vi "FR GUI Recalculate.vi"(11 "FFmeter settings":T1={"AC Source"={"AC Source type"=enum."Fluke 5XXX calibrator", "VISA"="", "Ref. clock (Hz)"=0.0, "status ref"=refnum}, "TWM pipe"="\\\\.\\pipe\\TWM:server", "Measurement status ref"=refnum, "TWM Status ref"=refnum, "Abort ref"=refnum, "DC meter"={"DC meter type"=enum."H/A/K 3458", "DC meter VISA"="", "NPLC"=10, "status ref"=refnum}, "Measurement properties"={"Measurement frequencies (Hz)"=[1000.0], "Sampling frequency (Hz)"=500000.0, "Signal amplitude (V)"=4.5, "AC-DC settle time (s)"=20.0, "Record length (multiples of period)"=[1000.0, 10000.0, 1000.0], "Measurement template file"=path "", "Row of START keyword"=0, "Row of STOP keyword"=0, "Calculate RMS from samples"=FALSE, "AC-DC warm up time (s)"=300.0, "Measurement template line"=[], "DC meter readings No."=10, "Algorithm"="TWM-WFFT", "Simultaneous measurement"=FALSE}, "Skip waiting ref"=refnum, "Octave paths"={"GNU Octave path"=path "C:/Program Files/GNU Octave/Octave-6.2.0/mingw64/bin", "TWM+QWTB path"=path "C:/Users/labina/Desktop/TWM-1.8.7.0-full/octprog", "lvlib path"=path "D:/martin/WAC/WACsw - github/control_software/Filter function meter/external libraries/GOLPI 0.7.3.1 source distribution LV 20.0 32 bit/lv_proc.dll"}, "Template definition"={"Keywords column"=0, "Sig. freq. column"=1, "Rec. len. column"=2, "Meas. points. row min to read"=9, "Meas. points. row max to read"=1509, "Properties column"=4, "Properties row start"=1, "Properties row end"=5, "Keyword START regexp"="", "Keyword STOP regexp"="", "HW data column"=7, "HW data row start"=1, "HW data row end"=3, "TIme and date column start"=3, "Digitizer value column start "=4, "DC mean column start "=6, "DC readings column start"=10}} {"Measurement properties"."Record length (multiples of period)" format="%#_3p"; "Measurement properties"."Sampling frequency (Hz)" format="%#_3p"; "Measurement properties"."Measurement frequencies (Hz)" format="%#_3p"}) -> (3 "FFmeter settings out":T1={"AC Source"={"AC Source type"=enum."Fluke 5XXX calibrator", "VISA"="", "Ref. clock (Hz)"=0.0, "status ref"=refnum}, "TWM pipe"="\\\\.\\pipe\\TWM:server", "Measurement status ref"=refnum, "TWM Status ref"=refnum, "Abort ref"=refnum, "DC meter"={"DC meter type"=enum."H/A/K 3458", "DC meter VISA"="", "NPLC"=10, "status ref"=refnum}, "Measurement properties"={"Measurement frequencies (Hz)"=[1000.0], "Sampling frequency (Hz)"=500000.0, "Signal amplitude (V)"=4.5, "AC-DC settle time (s)"=20.0, "Record length (multiples of period)"=[1000.0, 10000.0, 1000.0], "Measurement template file"=path "", "Row of START keyword"=0, "Row of STOP keyword"=0, "Calculate RMS from samples"=FALSE, "AC-DC warm up time (s)"=300.0, "Measurement template line"=[], "DC meter readings No."=10, "Algorithm"="TWM-WFFT", "Simultaneous measurement"=FALSE}, "Skip waiting ref"=refnum, "Octave paths"={"GNU Octave path"=path "C:/Program Files/GNU Octave/Octave-6.2.0/mingw64/bin", "TWM+QWTB path"=path "C:/Users/labina/Desktop/TWM-1.8.7.0-full/octprog", "lvlib path"=path "D:/martin/WAC/WACsw - github/control_software/Filter function meter/external libraries/GOLPI 0.7.3.1 source distribution LV 20.0 32 bit/lv_proc.dll"}, "Template definition"={"Keywords column"=0, "Sig. freq. column"=1, "Rec. len. column"=2, "Meas. points. row min to read"=9, "Meas. points. row max to read"=1509, "Properties column"=4, "Properties row start"=1, "Properties row end"=5, "Keyword START regexp"="", "Keyword STOP regexp"="", "HW data column"=7, "HW data row start"=1, "HW data row end"=3, "TIme and date column start"=3, "Digitizer value column start "=4, "DC mean column start "=6, "DC readings column start"=10}} {"Measurement properties"."Record length (multiples of period)" format="%#_3p"; "Measurement properties"."Sampling frequency (Hz)" format="%#_3p"; "Measurement properties"."Measurement frequencies (Hz)" format="%#_3p"})   [LabVIEW 2020]
doc: "Use this template to build a producer/consumer design pattern with events to produce queue items. Use this design pattern instead of the User Interface Event Handler pattern for user interfaces when you want to execute code asynchronously in response to an event without slowing the user interface responsiveness."
uses:
  Type definitions/FFmeter settings.ctl
  General AC source/Type definitions/AC Source.ctl
  General AC source/Type definitions/AC Source type.ctl
  General DC meter/Type definitions/DC meter.ctl
  General DC meter/Type definitions/DC meter type.ctl
  FR Measurement/Type definitions/FR Measuement properties.ctl
  FR Utilities/Type definitions/FR Template definition.ctl
  <vilib>/Utility/NIReport.llb/Report Type.ctl
  external libraries/GOLPI 0.7.3.1 source distribution LV 20.0 32 bit/GOLPI reference Type Def.ctl
  external libraries/GOLPI 0.7.3.1 source distribution LV 20.0 32 bit/Pipe Handle.ctl
  <vilib>/Utility/error.llb/Error Cluster From Error Code.vi
  <vilib>/addons/_office/excel.llb/Excel Get Data ([str]).vi
  <vilib>/ErrorRing/Error Ring.xnode
  <vilib>/Utility/NIReport.llb/NI_report.lvclass
  external libraries/varilib/varilib.lvlib
  <vilib>/addons/_office/NI_ReportGenerationToolkit.lvlib
  <vilib>/Utility/NIReport.llb/NI_ReportGenerationCore.lvlib
  external libraries/GOLPI 0.7.3.1 source distribution LV 20.0 32 bit/LV Process library.lvlib
  external libraries/GOLPI 0.7.3.1 source distribution LV 20.0 32 bit/GOLPI library.lvlib
  <vilib>/Utility/NIReport.llb/Excel/NI_Excel.lvclass
panel:
  out "template file":string
  in  "Abort":bool
  in  "skip calculated":bool caption="Skip already calculated (only rereads results)"
  out "Progress":i32(slide) min=0 max=266 scale=0.0..10.0
  in  "TWM+QWTB path":path=path "C:/Users/labina/Desktop/TWM-1.8.7.0-full/octprog"
  in  "GNU Octave path":path=path "C:/Program Files/GNU Octave/Octave-6.2.0/mingw64/bin"
  out "gui_elements":refnum<vi>[](array[refnum])
  in  "OK":bool
  in  "cancel":bool
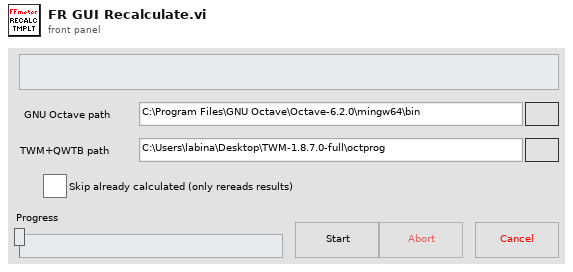
[diagram p1: front panel]
types:
  T1 = typedef "FFmeter settings.ctl" = cluster{"AC Source":T2, "TWM pipe":string, "Measurement status ref":refnum<vi>, "TWM Status ref":refnum<vi>, "Abort ref":refnum<vi>, "DC meter":T4, "Measurement properties":T6, "Skip waiting ref":refnum<vi>, "Octave paths":cluster{"GNU Octave path":path, "TWM+QWTB path":path, "lvlib path":path}, "Template definition":T7}
  T2 = typedef "AC Source.ctl" = cluster{"AC Source type":T3, "VISA":refnum<visa-resource-name>, "Ref. clock (Hz)":dbl, "status ref":refnum<vi>}
  T3 = typedef "AC Source type.ctl" = enum16{"Fluke 5XXX calibrator", "Tektronix AFG3000 series", "dummy"}
  T4 = typedef "DC meter.ctl" = cluster{"DC meter type":T5, "DC meter VISA":refnum<visa-resource-name>, "NPLC":i32, "status ref":refnum<vi>}
  T5 = typedef "DC meter type.ctl" = enum16{"H/A/K 3458", "Fluke 8508A", "dummy", "Keithley 2182"}
  T6 = typedef "FR Measuement properties.ctl" = cluster{"Measurement frequencies (Hz)":dbl[], "Sampling frequency (Hz)":dbl, "Signal amplitude (V)":dbl, "AC-DC settle time (s)":dbl, "Record length (multiples of period)":dbl[], "Measurement template file":path, "Row of START keyword":i32, "Row of STOP keyword":i32, "Calculate RMS from samples":bool, "AC-DC warm up time (s)":dbl, "Measurement template line":i32[], "DC meter readings No.":i32, "Algorithm":string, "Simultaneous measurement":bool}
  T7 = typedef "FR Template definition.ctl" = cluster{"Keywords column":i32, "Sig. freq. column":i32, "Rec. len. column":i32, "Meas. points. row min to read":i32, "Meas. points. row max to read":i32, "Properties column":i32, "Properties row start":i32, "Properties row end":i32, "Keyword START regexp":string, "Keyword STOP regexp":string, "HW data column":i32, "HW data row start":i32, "HW data row end":i32, "TIme and date column start":i32, "Digitizer value column start ":i32, "DC mean column start ":i32, "DC readings column start":i32}
  T8 = enum8{"Enabled", "Disabled", "Disabled and Grayed Out"}
  T9 = typedef "GOLPI library.lvlib/GOLPI reference Type Def.ctl" = cluster{"pipe handle":T10, "fast read timeout [ms]":u32, "fast read settle time [ms]":u32, "fast read to multiple [ms]":u32, "max elements per input line":u32, "slow read timeout [ms]":u32, "stdin double format specifier":string, "max elements per stdout output column":u32, "console mode bitstream":bool, "bitstream first read timeout [ms]":u32, "bitstream read timeout [ms]":u32, "struct transfer possible":bool, "matlab mode":bool}
  T10 = typedef "LV Process library.lvlib/Pipe Handle.ctl" = cluster{"lv_proc.dll file path":path, "process instance handle":u32[], "debug mode":bool, "debug data":cluster{"time":timestamp, "stdin":bool, "data":string}[]}
  T11 = enum16{"maximized", "minimized", "normal", "no change"}
  T12 = typedef "NI_ReportGenerationCore.lvlib/Report Type.ctl" = enum16{"HTML", "Word", "Excel"}
  T13 = cluster{"GNU Octave path":path, "TWM+QWTB path":path, "lvlib path":path}
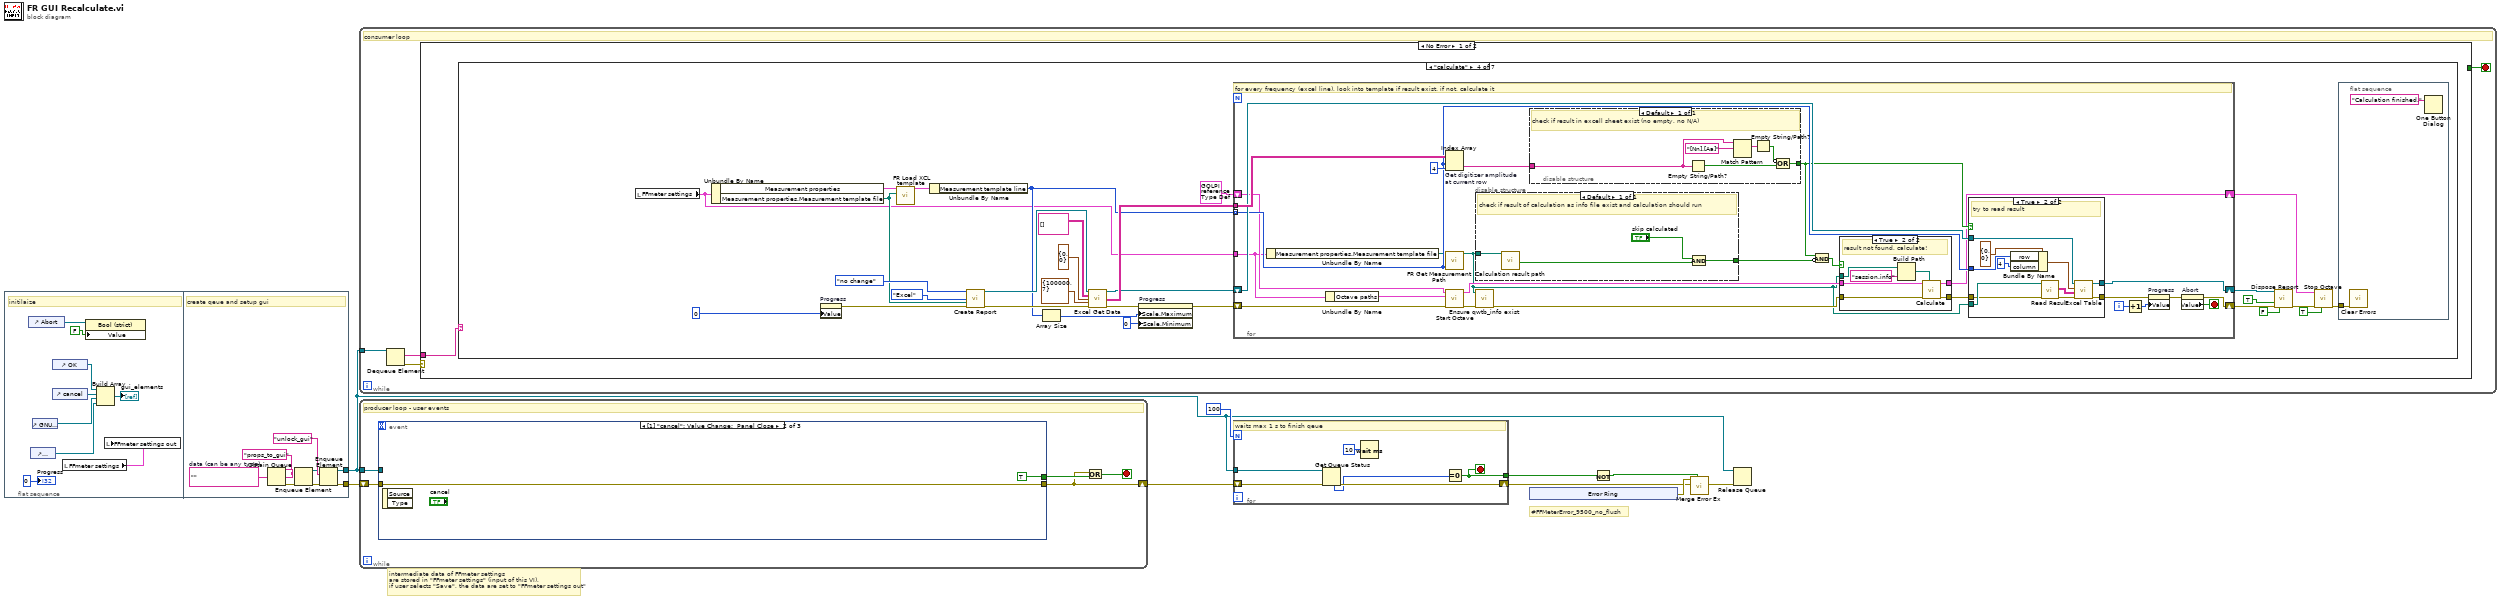
[diagram p0: block diagram]
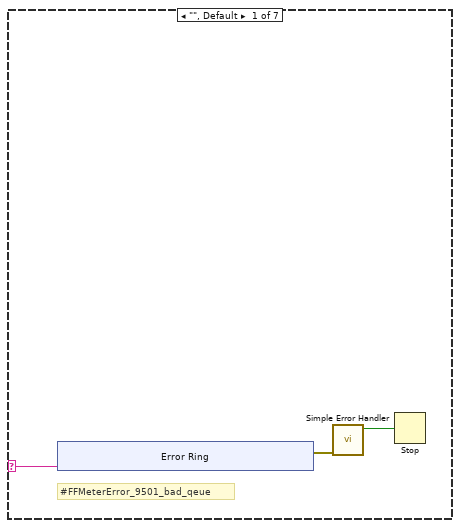
[diagram p2: hidden frame]
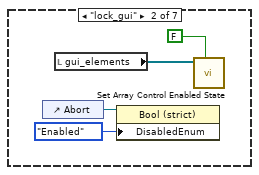
[diagram p3: hidden frame]
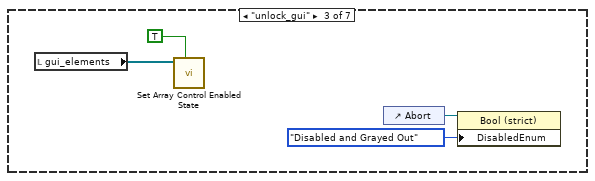
[diagram p4: hidden frame]
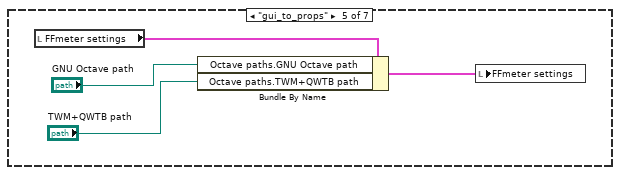
[diagram p7: hidden frame]
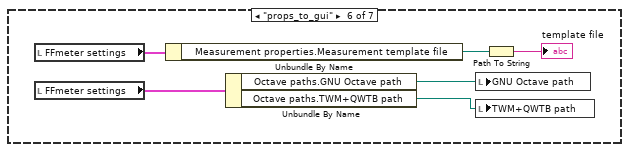
[diagram p8: hidden frame]
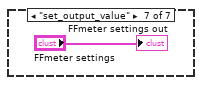
[diagram p9: hidden frame]
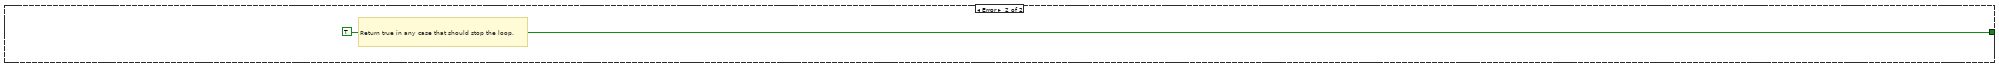
[diagram p10: hidden frame]
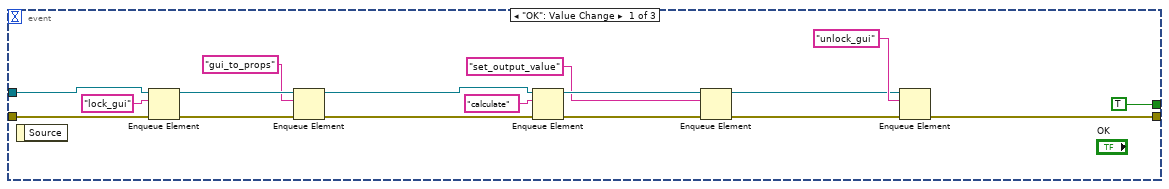
[diagram p11: hidden frame]
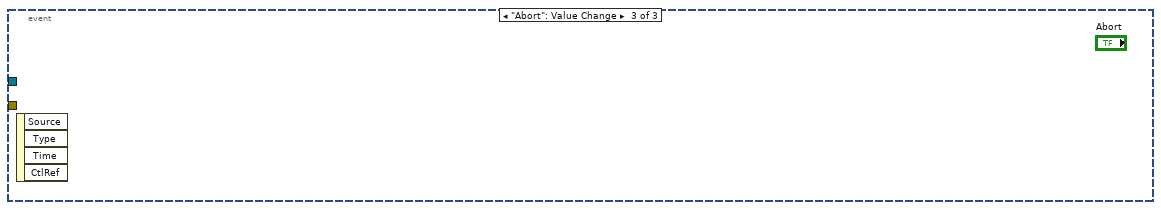
[diagram p12: hidden frame]
diagram:
  # "intermediate data of FFmeter settings\nare stored in \"FFmeter settings\" (input of this VI),\nif user selects \"Save\", the data are set to \"FFmeter settings out\""
  # "#FFMeterError_9500_no_flush"
  n1 = flat-sequence {
    tunnel: [w26] -> w2
    tunnel: [w24] -> w1
    frame #0 {
      # "initilaize"
      n2 = control-ref of="Abort"() -> (w12:refnum<vi>)
      n3 = control-ref of="TWM+QWTB path"() -> (w14:refnum<vi>)
      n4 = control-ref of="GNU Octave path"() -> (w15:refnum<vi>)
      n5 = control-ref of="OK"() -> (w18:refnum<vi>)
      n6 = control-ref of="cancel"() -> (w17:refnum<vi>)
      n7 = local read "FFmeter settings"() -> (w10:T1)
      n8 = property class="Bool (strict)"(reference=w12, "Value"=FALSE) -> ()  [unwired: 1 in, 2 out]
      n9 = Build Array(w18, w17, w15, w14) -> (→"gui_elements":refnum<vi>[])
      n10 = local write "FFmeter settings out"(w10) -> ()
      "Progress" <- 0 ("Progress")
    }
    frame #1 {
      w25 = ""  # data (can be any type)
      # "create qeue and setup gui"
      n11 = Obtain Queue(element data type=w25) -> (queue out=w21:refnum<queue>, error out=w20:errorcluster)  [unwired: 4 in, 1 out]
      n12 = Enqueue Element(queue=w21, element="props_to_gui", error in (no error)=w20) -> (queue out=w22:refnum<queue>, error out=w23:errorcluster)  [unwired: 1 in, 1 out]
      n13 = Enqueue Element(queue=w22, element="unlock_gui", error in (no error)=w23) -> (queue out=w26:refnum<queue>, error out=w24:errorcluster)  [unwired: 1 in, 1 out]
    }
  }
  n14 = while {
    tunnel: w2 -> [w31]
    stop <- w28 stop-if-true
    # "consumer loop"
    n15 = Dequeue Element(queue=w31) -> (element=w29:string, error out=w30:errorcluster)  [unwired: 2 in, 2 out]
    n16 = case shown="No Error" w30 {
      tunnel: w29 -> [w32 _]
      tunnel: [_ TRUE] -> w28
      frame No Error {
        n17 = case shown="\"calculate\"" w32 {
          selector: w32 -> [w33 _ _ _ _ _ _]
          frame "", Default {
            # "#FFMeterError_9501_bad_qeue"
            n18 = xnode "Error Ring"("parameter 0"=w33) -> ("error out"=w35:errorcluster)
            n19 = call <vilib>:"Simple Error Handler.vi"("error in (no error)"=w35) -> ("error?"=w34:bool)  [unwired: 4 in, 4 out]
            n20 = Stop(stop? (T)=w34) -> ()
          }
          frame "lock_gui" {
            n21 = control-ref of="Abort"() -> (w44:refnum<vi>)
            n22 = local read "gui_elements"() -> (w46:refnum<vi>[])
            n23 = property class="Bool (strict)"(reference=w44, "DisabledEnum"=T8."Enabled" ("Disabled")) -> ()  [unwired: 1 in, 2 out]
            n24 = call "Set Array Control Enabled State.vi"("enabled (T)"=FALSE, "reference array in"=w46) -> ()  [unwired: 8 in, 2 out]
          }
          frame "unlock_gui" {
            n25 = local read "gui_elements"() -> (w50:refnum<vi>[])
            n26 = call "Set Array Control Enabled State.vi"("enabled (T)"=TRUE, "reference array in"=w50) -> ()  [unwired: 8 in, 2 out]
            n27 = control-ref of="Abort"() -> (w47:refnum<vi>)
            n28 = property class="Bool (strict)"(reference=w47, "DisabledEnum"=T8."Disabled and Grayed Out" ("Disabled")) -> ()  [unwired: 1 in, 2 out]
          }
          frame "calculate" {
            n29 = local read "FFmeter settings"() -> (w62:T1)
            n30 = Unbundle By Name(w62) -> ("Measurement properties"=w72:T6, "Measurement properties.Measurement template file"=w69:path)
            n31 = property on="Progress" class="Slide (strict)"("Value"=0 ("Progress")) -> (error out=w66:errorcluster)  [unwired: 2 in, 1 out]
            n32 = call "FR Load XCL template.vi"("Measurement template file"=w69, "Measurement properties"=w72) -> ("Measurement properties out"=w71:T6)  [unwired: 9 in]
            n33 = Unbundle By Name(w71) -> ("Measurement template line"=w68:i32[])
            n34 = call <vilib>:"Create Report.vi"("window state (normal)"=T11."no change", "report type"=Report_Type."Excel", "template (empty)"=w69, "error in (no error)"=w66) -> ("report out"=w73:refnum<class "NI_report.lvclass">, "error out"=w74:errorcluster)  [unwired: 10 in]
            n35 = Array Size(array=w68) -> (size(s)=w67:i32)
            n36 = call-poly <vilib>:"Excel Get Data.vi"("report in"=w73, "data type"=string[][] [], "start (-1, -1)"=cluster{"row":i32, "column":i32} {"row"=0, "column"=0}, "end (-1, -1)"=cluster{"row":i32, "column":i32} {"row"=100000, "column"=7}, "error in (no error)"=w74) -> ("report out"=w63:refnum<class "NI_report.lvclass">, "data"=w70:string[][], "error out"=w61:errorcluster)  [unwired: 8 in]
            n37 = property on="Progress" class="Slide (strict)"(error in=w61, "Scale.Maximum"=w67, "Scale.Minimum"=0 ("Data Entry Limits:Minimum")) -> (error out=w60:errorcluster)  [unwired: 1 in, 1 out]
            n38 = for {
              tunnel: w68 -> [w102] mode=indexing
              shift-right: [w82] -> w54
              shift-left: w60 -> [w99]
              tunnel: w70 -> [w107]
              shift-right: [w83] -> w56
              shift-left: T9 {"pipe handle"={"lv_proc.dll file path"=path "", "process instance handle"=[], "debug mode"=FALSE, "debug data"=[]}, "fast read timeout [ms]"=500, "fast read settle time [ms]"=10, "fast read to multiple [ms]"=1, "max elements per input line"=100, "slow read timeout [ms]"=5000, "stdin double format specifier"="%_16e", "max elements per stdout output column"=100, "console mode bitstream"=FALSE, "bitstream first read timeout [ms]"=1000, "bitstream read timeout [ms]"=50, "struct transfer possible"=FALSE, "matlab mode"=FALSE} ("GOLPI ref. out") -> [w101]
              shift-right: [w90] -> w55
              shift-left: w63 -> [w103]
              tunnel: w62 -> [w97]
              i -> [w104]
              stop <- w84 stop-if-true
              # "for every frequency (excel line), look into template if result exist. if not, calculate it"
              n39 = Unbundle By Name(w97) -> ("Measurement properties.Measurement template file"=w95:path)
              n40 = Unbundle By Name(w97) -> ("Octave paths"=w98:T13)
              n41 = Index Array "Get digitizer amplitude\nat current row"(array=w107, index (row)=w102, index (col)=4 ("disabled index (col)")) -> (element=w105:string)
              n42 = call "FR Get Measurement Path.vi"("Template line"=w102, "Measurement template file"=w95) -> ("Measurement path"=w87:path)  [unwired: 8 in, 1 out]
              n43 = call "Start Octave.vi"("error in (no error)"=w99, "Octave paths"=w98, "GOLPI ref. in"=w101) -> ("error out"=w94:errorcluster, "GOLPI ref. out"=w100:T9)  [unwired: 7 in]
              n44 = disable-structure shown="Default" {
                disable-tunnel: w87 -> [w124]
                disable-tunnel: [w121] -> w86
                frame Enabled {
                  # "check if result of calculation as info file exist and calculation should run"
                  n45 = call "Calculation result path.vi"("Measurement path"=w124) -> ("file exists?"=w122:bool)  [unwired: 9 in, 1 out]
                  n46 = Compound Arithmetic op=AND("skip calculated", w122) -> (w121:bool)
                }
              }
              n47 = call "Ensure qwtb_info exist.vi"("error in"=w94, "Measurement path"=w87) -> ("error out"=w93:errorcluster)  [unwired: 9 in]
              n48 = disable-structure shown="Default" {
                disable-tunnel: w105 -> [w138]
                disable-tunnel: [w134] -> w88
                frame Enabled {
                  # "check if result in excell sheet exist (no empty, no N/A)"
                  n49 = Empty String/Path?(string/path=w138) -> (empty?=w135:bool)
                  n50 = Match Pattern(string=w138, regular expression="[Nn].[Aa]") -> (match substring=w137:string)  [unwired: 1 in, 3 out]
                  n51 = Empty String/Path?(string/path=w137) -> (empty?=w136:bool)
                  n52 = Compound Arithmetic op=OR(invert w136, w135) -> (w134:bool)
                }
              }
              n53 = Compound Arithmetic op=AND(w88, invert w86) -> (w92:bool)
              n54 = case shown="True" w92 {
                tunnel: w93 -> [w125 w133]
                tunnel: [w126 w132] -> w83
                tunnel: w100 -> [w126 w131]
                tunnel: [w125 w130] -> w89
                tunnel: w87 -> [_ w128]
                frame False {
                  # "result existr"
                }
                frame True {
                  # "result not found, calculate!"
                  n55 = Build Path(base path=w128, name or relative path="session.info") -> (appended path=w127:path)
                  n56 = call "Calculate.vi"("Measurement path in"=w127, "error in (no error)"=w133, "GOLPI ref. in"=w131) -> ("error out"=w130:errorcluster, "GOLPI ref. out"=w132:T9)  [unwired: 7 in]
                }
              }
              n57 = case shown="True" w88 {
                tunnel: w103 -> [w108 w120]
                tunnel: w102 -> [_ w119]
                tunnel: w87 -> [_ w118]
                tunnel: [w109 w117] -> w91
                tunnel: [w108 w116] -> w90
                tunnel: w89 -> [w109 w112]
                frame False {
                }
                frame True {
                  # "try to read result"
                  n58 = Bundle By Name(cluster=cluster{"row":i32, "column":i32} {"row"=0, "column"=0} ("start (0, 0)"), "row"=w119, "column"=4) -> (w113:cluster{"row":i32, "column":i32})
                  n59 = call "Read Result.vi"("error in (no error)"=w112, "Measurement path"=w118) -> ("error out"=w111:errorcluster, "Result (val, unc)"=w110:string[][])  [unwired: 8 in]
                  n60 = call "Excel Table.vi"("error in (no error)"=w111, "table"=w110, "start (0, 0)"=w113, "report in"=w120) -> ("error out"=w117:errorcluster, "report out"=w116:refnum<class "NI_report.lvclass">)  [unwired: 6 in]
                }
              }
              n61 = Increment(x=w104) -> (x+1=w96:i32)
              n62 = property on="Progress" class="Slide (strict)"(error in=w91, "Value"=w96) -> (error out=w85:errorcluster)  [unwired: 1 in, 1 out]
              n63 = property on="Abort" class="Bool (strict)"(error in=w85) -> (error out=w82:errorcluster, "Value"=w84:bool)  [unwired: 1 in, 1 out]
            }
            n64 = call-dynamic "Dispose Report.vi"("report in"=w55, "save changes? (F)"=TRUE, "error in (no error)"=w54, "close report? (T)"=FALSE) -> ("error out"=w53:errorcluster)  [unwired: 11 in]
            n65 = call "Stop Octave.vi"("Stop Octave?"=TRUE, "error in (no error)"=w53, "GOLPI ref. in"=w56) -> ("error out"=w57:errorcluster)  [unwired: 7 in, 1 out]
            n66 = flat-sequence {
              tunnel: w57 -> [w80]
              frame #0 {
                n67 = call <vilib>:"Clear Errors.vi"("error in (no error)"=w80) -> ()  [unwired: 5 in, 2 out]
                n68 = One Button Dialog(message="Calculation finished.") -> ()  [unwired: 1 in, 1 out]
              }
            }
          }
          frame "gui_to_props" {
            n69 = local read "FFmeter settings"() -> (w143:T1)
            n70 = Bundle By Name(cluster=w143, "Octave paths.GNU Octave path"="GNU Octave path", "Octave paths.TWM+QWTB path"="TWM+QWTB path") -> (w142:T1)
            n71 = local write "FFmeter settings"(w142) -> ()
          }
          frame "props_to_gui" {
            n72 = local read "FFmeter settings"() -> (w145:T1)
            n73 = local read "FFmeter settings"() -> (w149:T1)
            n74 = Unbundle By Name(w145) -> ("Measurement properties.Measurement template file"=w146:path)
            n75 = Unbundle By Name(w149) -> ("Octave paths.GNU Octave path"=w147:path, "Octave paths.TWM+QWTB path"=w148:path)
            n76 = local write "GNU Octave path"(w147) -> ()
            n77 = local write "TWM+QWTB path"(w148) -> ()
            n78 = Path To String(path=w146) -> (string=→"template file":string)
          }
          frame "set_output_value" {
            "FFmeter settings out" <- "FFmeter settings"
          }
        }
      }
      frame Error {
        # "Return true in any case that should stop the loop."
      }
    }
  }
  n79 = while {
    shift-right: [w152] -> w5
    shift-left: w1 -> [w155]
    tunnel: w2 -> [w156]
    stop <- w153 stop-if-true
    # "producer loop - user events"
    n80 = event shown="[1] \"cancel\": Value Change;  Panel Close" {
      selector: _ -> [_ _ _]
      dyn-events: _ -> [_ _ _]
      timeout: _ -> [_ _ _]
      tunnel: w156 -> [w170 _ _]
      tunnel: w155 -> [w169 w175 _]
      tunnel: [w167 w175 _] -> w152
      tunnel: [TRUE ("cancel") TRUE ("cancel") _] -> w154
      event "OK": Value Change {
        n81 = event-data() -> ()  [unwired: 1 in, 1 out]
        n82 = Enqueue Element(queue=w170, element="lock_gui", error in (no error)=w169) -> (queue out=w163:refnum<queue>, error out=w166:errorcluster)  [unwired: 1 in, 1 out]
        n83 = Enqueue Element(queue=w163, element="gui_to_props", error in (no error)=w166) -> (queue out=w164:refnum<queue>, error out=w165:errorcluster)  [unwired: 1 in, 1 out]
        n84 = Enqueue Element(queue=w164, element="calculate", error in (no error)=w165) -> (queue out=w158:refnum<queue>, error out=w161:errorcluster)  [unwired: 1 in, 1 out]
        n85 = Enqueue Element(queue=w158, element="set_output_value", error in (no error)=w161) -> (queue out=w159:refnum<queue>, error out=w160:errorcluster)  [unwired: 1 in, 1 out]
        n86 = Enqueue Element(queue=w159, element="unlock_gui", error in (no error)=w160) -> (error out=w167:errorcluster)  [unwired: 1 in, 2 out]
      }
      event "cancel": Value Change; Panel Close {
        n87 = event-data() -> ()  [unwired: 1 in, 2 out]
      }
      event "Abort": Value Change {
        n88 = event-data() -> ()  [unwired: 1 in, 4 out]
      }
    }
    n89 = Or(x=w152, y=w154) -> (x .or. y?=w153:bool)
  }
  n90 = for {
    N: 100 -> [_]
    tunnel: w2 -> [w181]
    shift-right: [w179] -> w6
    shift-left: w5 -> [w180]
    tunnel: [w176] -> w3
    stop <- w176 stop-if-true
    # "waits max 1 s to finish qeue"
    n91 = Get Queue Status(queue=w181, error in (no error)=w180) -> (error out=w179:errorcluster, # elements in queue=w177:i32)  [unwired: 1 in, 6 out]
    n92 = Wait (ms)(milliseconds to wait=u32 10) -> ()  [unwired: 1 out]
    n93 = Equal To 0?(x=w177) -> (x = 0?=w176:bool)
  }
  n94 = xnode "Error Ring"() -> ("error out"=w7:errorcluster)
  n95 = Not(x=w3) -> (.not. x?=w8:bool)
  n96 = call "Merge Error Ex.vi"("Is error? (False)"=w8, "main error in (no error)"=w6, "second error in"=w7) -> ("error out"=w4:errorcluster)  [unwired: 8 in]
  n97 = Release Queue(queue=w2, error in (no error)=w4) -> ()  [unwired: 1 in, 3 out]
